vi "WebcamReadandShow.vi"() -> ()   [LabVIEW 2015]
uses:
  <vilib>/picture/picture.llb/imagedata.ctl
  <vilib>/httpClient/LabVIEWHTTPClient.lvlib
panel:
  in  "[user-specified font]":T1={"Font Name:"="Apple Casual", "Size"=26, "Strikeout?"=FALSE, "Italic?"=FALSE, "Underline?"=FALSE, "Outline?"=FALSE, "Shadow?"=FALSE, "Bold?"=TRUE}
  in  "desired font(Application)":T2(ring)
  in  "origin":cluster{"x":i16, "y":i16}={"x"=200, "y"=20}
  in  "text":string="TOAP too!"
  out "2D Picture":picture
  out "image data":T3={"image type"=0, "image depth"=24, "image"=array[921600 elements], "mask"=[], "colors"=[], "Rectangle"={"left"=0, "top"=0, "right"=640, "bottom"=480}}
  out "body":string
  out "headers":string="HTTP/1.0 200 OK\r\nExpires: -1\r\nCache-Control: no-cache\r\nContent-length: 42188\r\nContent-type: image/jpeg\r\n\r\n"
  in  "url":string="https://0.academia-photos.com/2842261/938572/1175579/s200_kerstin.enflo.jpg"
  # "Example webcams:Panasonics:\nhttp://wt1_cam.cppwind.local/SnapshotJPEG?Resolution=640x480\nhttp://wt3_cam.cppwind.local/SnapshotJPEG?Resolution=640x480\n\n(resolution is optionalÉ)"
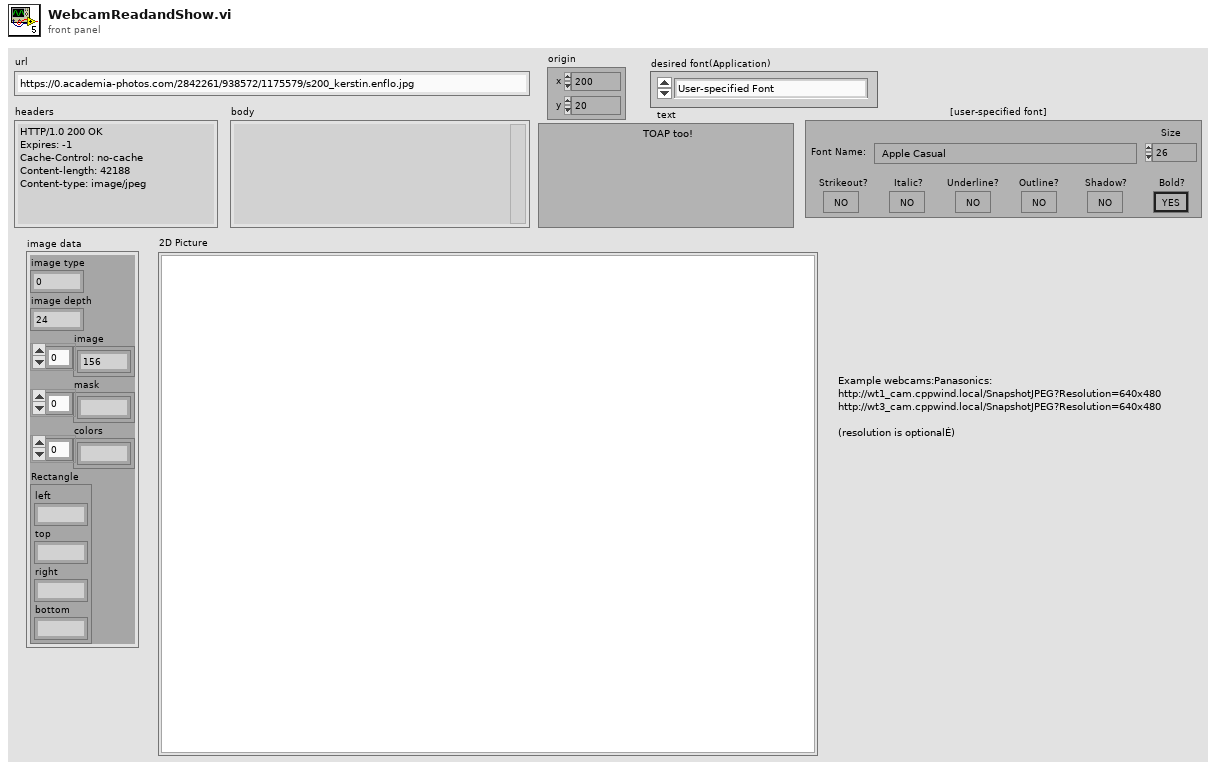
[diagram p1: front panel]
types:
  T1 = cluster{"Font Name:":string, "Size":i16, "Strikeout?":bool, "Italic?":bool, "Underline?":bool, "Outline?":bool, "Shadow?":bool, "Bold?":bool}
  T2 = enum16{"User-specified Font", "Application Font", "System Font", "Dialog Font"}
  T3 = typedef "imagedata.ctl" = cluster{"image type":i32, "image depth":i32, "image":u8[], "mask":u8[], "colors":u32[], "Rectangle":cluster{"left":i16, "top":i16, "right":i16, "bottom":i16}}
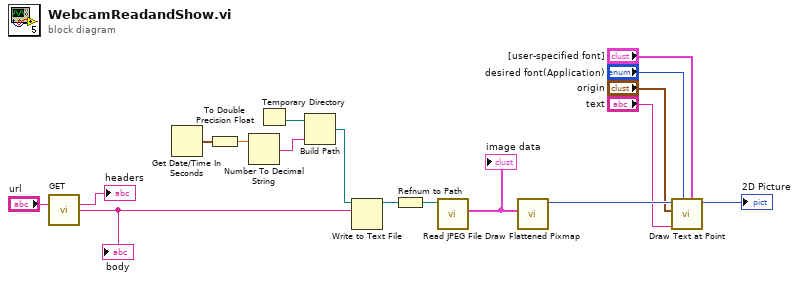
[diagram p0: block diagram]
diagram:
  n1 = call <vilib>:"GET.vi"("url"="url") -> ("headers"=→"headers":string, "body"=w15:string)  [unwired: 11 in, 2 out]
  "body" <- w15
  n2 = Get Date/Time In Seconds() -> (seconds since 1Jan1904=w3:timestamp)
  n3 = To Double Precision Float(number=w3) -> (double precision float=w2:dbl)
  n4 = Number To Decimal String(number=w2) -> (decimal integer string=w1:string)  [unwired: 1 in]
  n5 = Temporary Directory() -> (w4:path)
  n6 = Build Path(base path=w4, name or relative path=w1) -> (appended path=w5:path)
  n7 = Write to Text File(file (use dialog)=w5, text=w15) -> (refnum out=w14:refnum<file>)  [unwired: 2 in, 2 out]
  n8 = Refnum to Path(1:w14) -> (0:w13:path)
  n9 = call <vilib>:"Read JPEG File.vi"("path to JPEG file"=w13) -> ("image data"=w12:T3)  [unwired: 8 in, 2 out]
  "image data" <- w12
  n10 = call <vilib>:"Draw Flattened Pixmap.vi"("image data"=w12) -> ("new picture"=w11:picture)  [unwired: 8 in]
  n11 = call <vilib>:"Draw Text at Point.vi"("[user-specified font]"="[user-specified font]", "desired font(Application)"="desired font(Application)", "text"="text", "origin"="origin", "picture"=w11) -> ("new picture"=→"2D Picture":picture)  [unwired: 5 in, 1 out]
